vi "Stop.vi"(8 "error in (no error)":errorcluster) -> (0 "error out":errorcluster)   [LabVIEW 2017, in "BOP_VibAPI_8.lvlib"]
uses:
  <vilib>/addons/InsightCM/Devices/Shared/Cms/Fpga/Acquisition/source/subVIs/VibAPI_8/BOP_VibAPI_8.lvlib
  <vilib>/rvi/eio/common/nirviEmuTemplateMethod_errors.vi
  <vilib>/eio/EIONode/EIONode.xnode
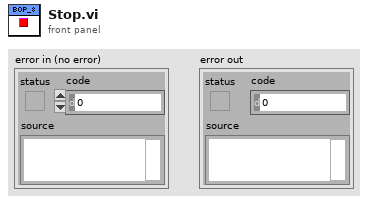
[diagram p1: front panel]
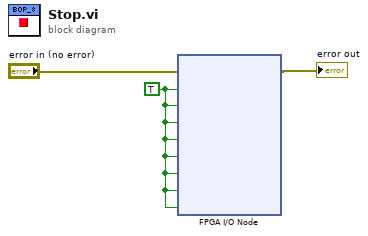
[diagram p0: block diagram]
diagram:
  w1 = TRUE ("Mod1/Stop")
  n1 = xnode "FPGA I/O Node"("error in"="error in (no error)", "Mod1/Stop"=w1, "Mod2/Stop"=w1, "Mod3/Stop"=w1, "Mod4/Stop"=w1, "Mod5/Stop"=w1, "Mod6/Stop"=w1, "Mod7/Stop"=w1, "Mod8/Stop"=w1) -> ("error out"=→"error out":errorcluster)  [unwired: 8 in, 8 out]
